vi "FTP_SendFile.vi"(0 "Remote Path":string, 1 "Admin?":bool=TRUE, 2 "file path (<NAP>)":path=path "", 3 "error in (no error)":errorcluster) -> (6 "Success?":bool, 7 "error out":errorcluster)   [LabVIEW 2012]
panel:
  out "OnServer?":bool
  out "CWD":bool
  out "STOR":bool
  out "type":bool
  out "pasv":bool
  out "closed":bool
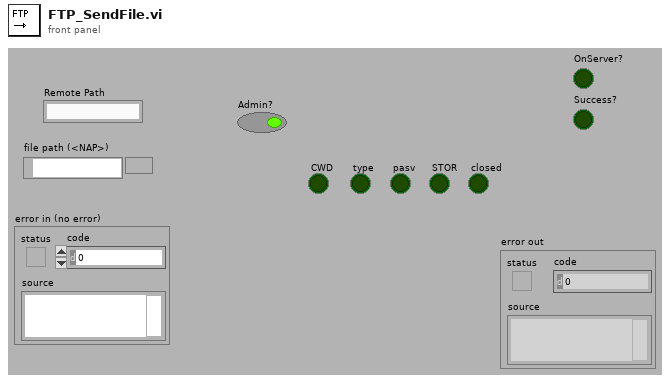
[diagram p1: front panel]
types:
  T1 = cluster{"passive address":string, "passive port":u16}
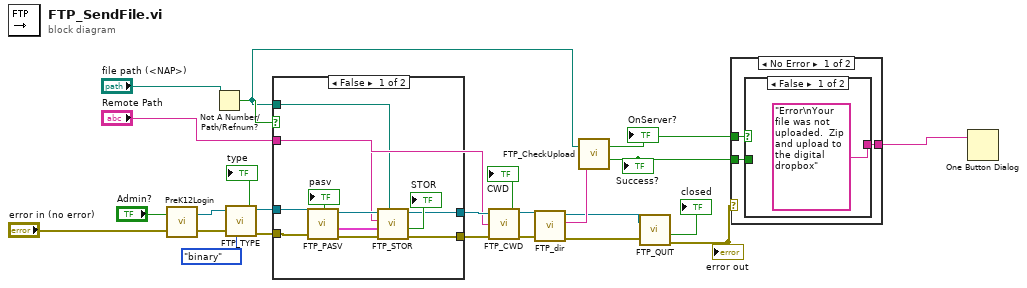
[diagram p0: block diagram]
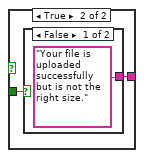
[diagram p2: hidden frame]
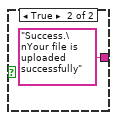
[diagram p3: hidden frame]
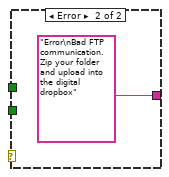
[diagram p4: hidden frame]
diagram:
  n1 = call <userlib>:"PreK12Login.vi"("error in (no error)"="error in (no error)", "Admin?"="Admin?") -> ("error out"=w16:errorcluster, "connection ID out"=w17:refnum<k5>)
  n2 = Not A Number/Path/Refnum?(number/path/refnum="file path (<NAP>)") -> (NaN/Path/Refnum?=w11:bool)
  n3 = call <userlib>:"FTP_TYPE.vi"("connection ID"=w17, "type (query)"=enum16{"(query)", "ASCII", "binary"}."binary", "error in"=w16) -> ("connection ID out"=w22:refnum<k5>, "Good Reply?"=→"type":bool, "error out"=w21:errorcluster)  [unwired: 1 out]
  n4 = case shown="False" w11 {
    tunnel: w22 -> [w32 w37]
    tunnel: w21 -> [w31 w36]
    tunnel: "file path (<NAP>)" -> [w29 _]
    tunnel: [w27 w37] -> w15
    tunnel: [w26 w36] -> w14
    tunnel: "Remote Path" -> [w25 _]
    frame False {
      n5 = call <userlib>:"FTP_PASV.vi"("connection ID"=w32, "error in"=w31) -> ("connection ID out"=w34:refnum<k5>, "Passive Port"=w30:T1, "Good Reply?"=→"pasv":bool, "error out"=w33:errorcluster)  [unwired: 1 out]
      n6 = call <userlib>:"FTP_STOR.vi"("file path"=w29, "error in"=w33, "Passive Port"=w30, "Remote Path"=w25, "connection ID"=w34) -> ("error out"=w26:errorcluster, "Good Reply?"=→"STOR":bool, "connection ID out"=w27:refnum<k5>)  [unwired: 1 in, 1 out]
    }
    frame True {
    }
  }
  n7 = call <userlib>:"FTP_CWD.vi"("connection ID"=w15, "path"="Remote Path", "error in"=w14) -> ("connection ID out"=w9:refnum<k5>, "Good Reply?"=→"CWD":bool, "error out"=w10:errorcluster)  [unwired: 1 out]
  n8 = call <userlib>:"FTP_dir.vi"("connection ID"=w9, "error in"=w10) -> ("connection ID out"=w2:refnum<k5>, "reply string"=w7:string, "error out"=w1:errorcluster)  [unwired: 2 out]
  n9 = call <userlib>:"FTP_CheckUpload.vi"("reply string"=w7, "file path (<NAP>)"="file path (<NAP>)") -> ("same size?"=w4:bool, "On server?"=w5:bool)
  "Success?" <- w4
  "OnServer?" <- w5
  n10 = call <userlib>:"FTP_QUIT.vi"("connection ID"=w2, "error in"=w1) -> ("Good Reply?"=→"closed":bool, "error out"=w6:errorcluster)  [unwired: 2 out]
  "error out" <- w6
  n11 = case shown="No Error" w6 {
    tunnel: w5 -> [w40 _]
    tunnel: w4 -> [w39 _]
    tunnel: [w38 "Error\nBad FTP communication.  Zip your folder and upload into the digital dropbox"] -> w3
    frame No Error {
      n12 = case shown="False" w40 {
        tunnel: w39 -> [_ w43]
        tunnel: ["Error\nYour file was not uploaded.  Zip and upload to the digital dropbox" w42] -> w38
        frame False {
        }
        frame True {
          n13 = case shown="False" w43 {
            tunnel: ["Your file is uploaded successfully but is not the right size." "Success.\nYour file is uploaded successfully"] -> w42
            frame False {
            }
            frame True {
            }
          }
        }
      }
    }
    frame Error {
    }
  }
  n14 = One Button Dialog(message=w3) -> ()  [unwired: 2 out]
